vi "init zeromq vi.vi"(8 "error in (no error)":errorcluster, 11 "Server in":refnum<class "Server.lvclass">) -> (0 "error out":errorcluster, 3 "Server out":refnum<class "Server.lvclass">)   [LabVIEW 2018, in "Server.lvclass"]
uses:
  Server.lvclass
  Server.lvclass/Server.ctl
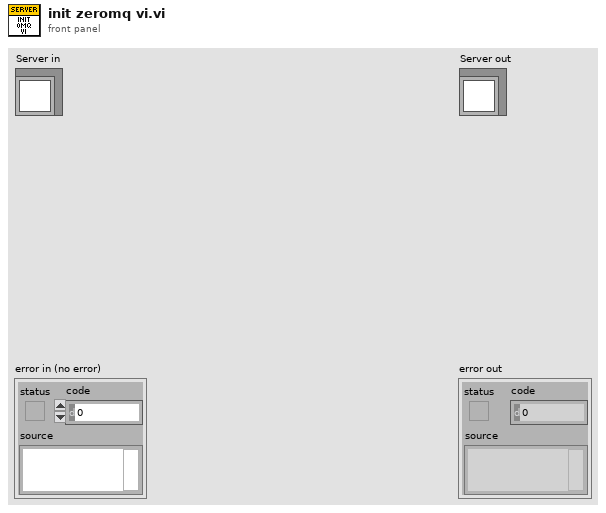
[diagram p1: front panel]
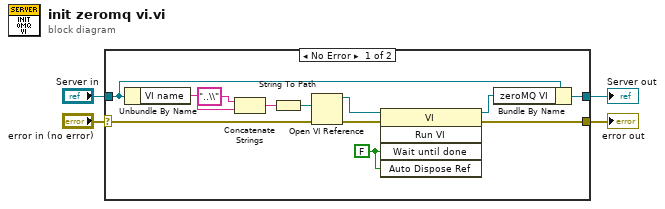
[diagram p0: block diagram]
diagram:
  n1 = case shown="No Error" "error in (no error)" {
    selector: "error in (no error)" -> [w10 w18]
    tunnel: [w9 w18] -> w3
    tunnel: [w8 w17] -> w1
    tunnel: "Server in" -> [w6 w17]
    frame No Error {
      w15 = FALSE ("Wait Until Done")
      n2 = Unbundle By Name(w6) -> ("VI name"=w5:string)
      n3 = Concatenate Strings("..\\", w5) -> (w12:string)
      n4 = String To Path(string=w12) -> (path=w14:path)
      n5 = Open VI Reference(vi path=w14, error in (no error)=w10) -> (vi reference=w16:refnum<vi>, error out=w13:errorcluster)  [unwired: 4 in]
      n6 = invoke class="VI" method="Run VI"(reference=w16, error in=w13, "Wait until done"=w15, "Auto Dispose Ref"=w15) -> (reference out=w7:refnum<vi>, error out=w9:errorcluster)  [unwired: 1 in, 3 out]
      n7 = Bundle By Name(cluster=w6, "zeroMQ VI"=w7) -> (w8:refnum<class "Server.lvclass">)
    }
    frame Error {
    }
  }
  "error out" <- w3
  "Server out" <- w1
